vi "陀螺仪.vi"() -> ()   [LabVIEW 2017]
uses:
  <vilib>/myRIO/Instrument Drivers/Onboard IO/I2C/typedefs/I2C User Configuration.ctl
  <vilib>/myRIO/Instrument Drivers/Onboard IO/I2C/typedefs/I2C Transfer Rate.ctl
  <vilib>/Platform/TimedLoop/XDataNode/timing_clust.ctl
  <vilib>/Platform/TimedLoop/XDataNode/nitl_modes.ctl
  <vilib>/Platform/TimedLoop/XDataNode/wakeup.ctl
  <vilib>/myRIO/Instrument Drivers/Onboard IO/I2C/typedefs/I2C Reference.ctl
  <vilib>/myRIO/Common/Instrument Driver Framework/Utilities/typedefs/myRIO Generic Hardware Reference.ctl
  <vilib>/myRIO/Common/Instrument Driver Framework/Utilities/typedefs/Hardware Version Enum.ctl
  <vilib>/myRIO/Common/Instrument Driver Framework/Utilities/typedefs/myRIO v1.0 Reference.ctl
  <vilib>/myRIO/Common/Instrument Driver Framework/Utilities/typedefs/Generic FPGA Reference.ctl
  <vilib>/myRIO/Common/Instrument Driver Framework/myRIO v1.0/I2C/typedefs/I2C Channels Enum.ctl
  <vilib>/myRIO/Instrument Drivers/Onboard IO/I2C/typedefs/I2C Configuration.ctl
  <vilib>/userdefined/High Color/nirio_resource_hc.ctl
  <vilib>/myRIO/Common/Instrument Driver Framework/myRIO v1.0/I2C/vis/myRIO v1.1 Open I2C.vi
  <vilib>/myRIO/Common/Instrument Driver Framework/Utilities/vis/Validate Channels.vi
  <vilib>/myRIO/Common/Instrument Driver Framework/myRIO v1.0/I2C/vis/myRIO v1.0 Reserve I2C.vi
  <vilib>/myRIO/Common/Instrument Driver Framework/myRIO v1.0/UART/vis/myRIO v1.0 Close UART.vi
  <vilib>/myRIO/Common/Instrument Driver Framework/myRIO v1.0/I2C/vis/myRIO v1.0 Build MUX Configuration I2C.vi
  <vilib>/myRIO/Common/Instrument Driver Framework/myRIO v1.0/Resource Manager/vis/myRIO v1.0 Reserve Channel List.vi
  <vilib>/myRIO/Common/Instrument Driver Framework/myRIO v1.0/Resource Manager/vis/myRIO v1.0 Create Configuration List.vi
  <vilib>/myRIO/Common/Instrument Driver Framework/myRIO v1.0/Resource Manager/vis/myRIO v1.0 Reserve Channel.vi
  <vilib>/myRIO/Common/Instrument Driver Framework/myRIO v1.0/Resource Manager/vis/myRIO v1.0 Unreserve Channel.vi
  <vilib>/myRIO/Common/Instrument Driver Framework/myRIO v1.0/Resource Manager/vis/myRIO v1.0 Build Mutex Name.vi
  <vilib>/Utility/VariantDataType/GetNumericInfo.vi
  <vilib>/Utility/error.llb/Error Cluster From Error Code.vi
  <vilib>/myRIO/Common/Instrument Driver Framework/myRIO v1.0/myRIO v1.1 Open.vi
  <vilib>/myRIO/Common/Instrument Driver Framework/Utilities/vis/IO Manager.vi
  <vilib>/myRIO/Common/Instrument Driver Framework/Utilities/vis/Configuration Manager.vi
  <vilib>/myRIO/Common/Instrument Driver Framework/myRIO v1.0/Resource Manager/vis/myRIO v1.0 Configure IO.vi
  <vilib>/myRIO/Common/Instrument Driver Framework/myRIO v1.0/myRIO v1.0 Close.vi
  <vilib>/myRIO/Common/Instrument Driver Framework/myRIO v1.0/I2C/vis/myRIO v1.0 Configure I2C.vi
  <vilib>/myRIO/Common/Instrument Driver Framework/myRIO v1.0/I2C/vis/myRIO v1.0 Write I2C.vi
  <vilib>/myRIO/Common/Instrument Driver Framework/myRIO v1.0/I2C/vis/myRIO v1.0 Read I2C.vi
  <vilib>/myRIO/Common/Instrument Driver Framework/Utilities/vis/FPGA Ref Manager.vi
  <vilib>/myRIO/Common/Instrument Driver Framework/myRIO v1.0/myRIO v1.0 Reset FPGA.vi
  <vilib>/myRIO/Common/Instrument Driver Framework/myRIO v1.0/IRQ/vis/myRIO v1.0 IRQ Info FGV.vi
  <vilib>/myRIO/Common/Instrument Driver Framework/myRIO v1.0/IRQ/vis/myRIO v1.0 Timer IRQ Info FGV.vi
  <vilib>/myRIO/Common/Instrument Driver Framework/myRIO v1.0/IRQ/vis/myRIO v1.0 ISR Agent.vi
  <vilib>/myRIO/Instrument Drivers/Onboard IO/I2C/vis/myRIO I2C Open.xnode
  <vilib>/Platform/TimedLoop/XDataNode/XDataNode.xnode
  <vilib>/myRIO/Instrument Drivers/Onboard IO/I2C/I2C.lvlib
  <vilib>/ptbypt/NI_PtbyPt.lvlib
  <vilib>/Platform/TimedLoop/XDataNode/XDNodeRunTimeDep.lvlib
  <vilib>/myRIO/Instrument Drivers/Utilities/Utilities.lvlib
panel:
  in  "y":dbl=26.5
  in  "x":dbl=-16.0
  in  "initialize":bool caption="初始化"
  in  "停止":bool
  out "加速度":cluster{i16, i16, i16}(graph)
  out "角度":T1(graph)
  out "角速度":cluster{"x":dbl, dbl, dbl}(graph)
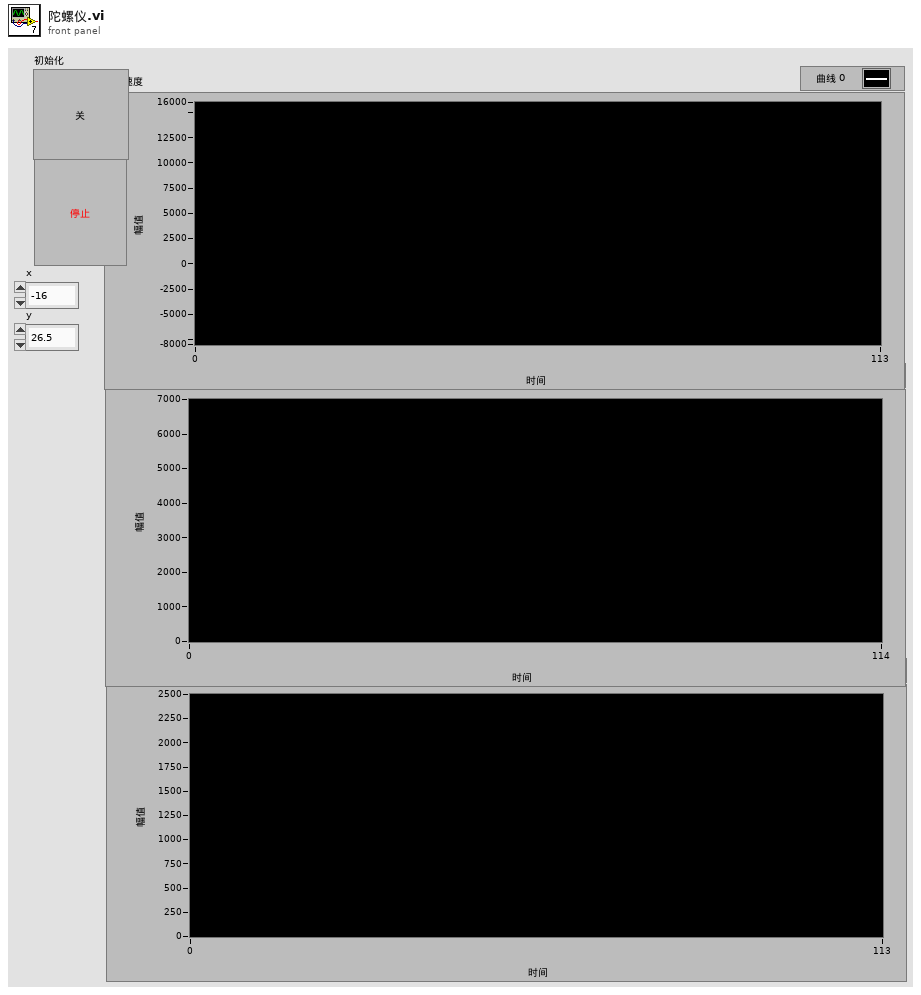
[diagram p1: front panel]
types:
  T1 = cluster{"integral x(t)":dbl, "integral x(t)":dbl, "integral x(t)":dbl}
  T2 = typedef "I2C.lvlib/I2C User Configuration.ctl" = cluster{"I2C Transfer Rate":T3}
  T3 = typedef "I2C.lvlib/I2C Transfer Rate.ctl" = enum16{"Standard mode (100 kbps)", "Fast mode (400 kbps)"}
  T4 = typedef "I2C.lvlib/I2C Reference.ctl" = cluster{"myRIO Reference":T5, "I2C Channels Enum":T9, "I2C Configuration":T10}
  T5 = typedef "myRIO Generic Hardware Reference.ctl" = cluster{"myRIO Model":T6, "myRIO Hardware Reference":T7}
  T6 = typedef "Hardware Version Enum.ctl" = enum16{"Unknown", "myRIO-1900", "myRIO-1950", "roboRIO", "NI ELVIS RIO CM"}
  T7 = typedef "myRIO v1.0 Reference.ctl" = cluster{"Generic FPGA Reference":T8, "Allow multiple opens":bool}
  T8 = typedef "Generic FPGA Reference.ctl" = refnum<k20>
  T9 = typedef "I2C Channels Enum.ctl" = enum16{"Not Connected", "A/I2C", "B/I2C", "I2C/I2C"}
  T10 = typedef "I2C.lvlib/I2C Configuration.ctl" = cluster{"I2C Transfer Rate":T3}
  T11 = typedef "XDNodeRunTimeDep.lvlib/timing_clust.ctl" = cluster{"Expected End [f-1]":u64, "Actual End [f-1]":u64, "Finished Late? [f-1]":bool, "Expected End [i-1]":u64, "Actual End [i-1]":u64, "Finished Late? [i-1]":bool, "Expected Start [i]":u64, "Actual Start [i]":u64, "Expected Start [f]":u64, "Actual Start [f]":u64, "Source Name":string, "Structure Name":string, "Period":i64, "Deadline":i64, "Offset":i64, "Start":i64, "Priority":i32, "Timeout":i32, "Mode":T12, "Wakeup Reason":T13, "Error":errorcluster, "Source Type":string, "Secondary Source Type":string, "Global End Time":u64, "Global Start Time":u64, "Frame Duration":u64, "Iteration Duration":u64, "Assigned CPU":i32, "I/O Scan Engine Mode":u32}
  T12 = typedef "XDNodeRunTimeDep.lvlib/nitl_modes.ctl" = enum32{"No Change", "Process missed periods, maintain original phase", "Discard missed periods, maintain original phase", "Process missed periods, ignore original phase", "Discard missed periods, ignore original phase"}
  T13 = typedef "XDNodeRunTimeDep.lvlib/wakeup.ctl" = enum32{"Normal", "Aborted", "Asynchronous wakeup", "Timing source error", "Timed loop error", "Timeout"}
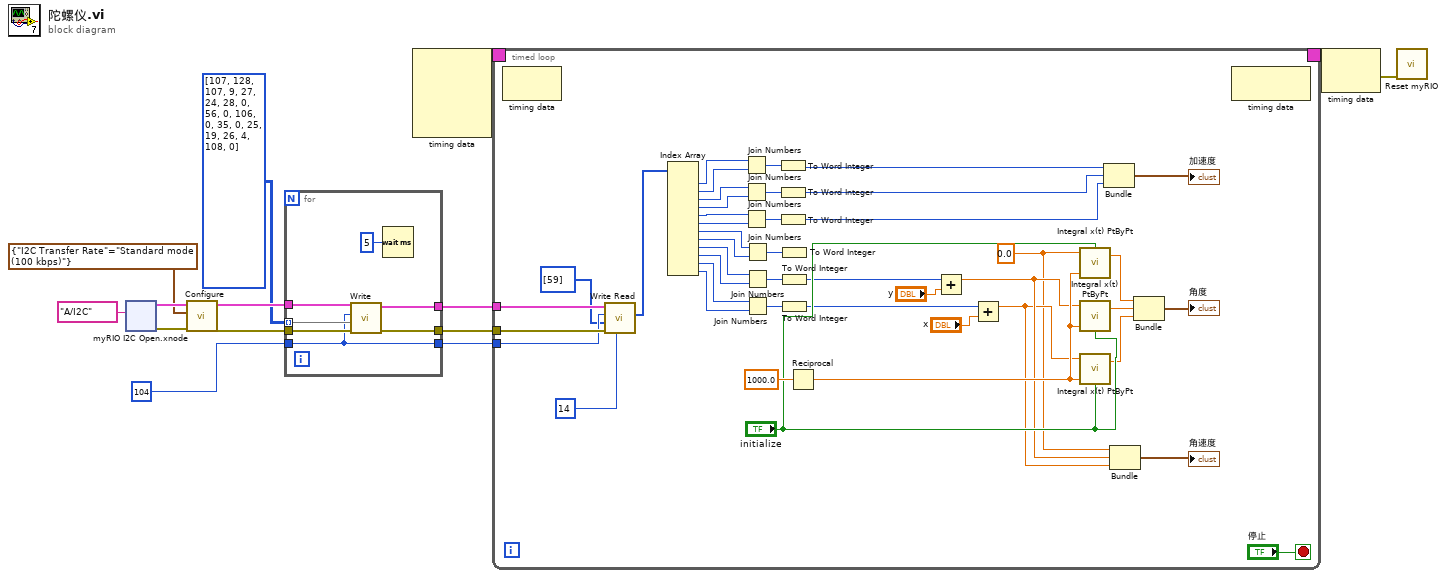
[diagram p0: block diagram]
diagram:
  n1 = xnode "myRIO I2C Open.xnode"("Channel Name"=tag "A/I2C") -> ("error out"=w14:errorcluster, "I2C Ref Out"=w13:T4)  [unwired: 2 in]
  n2 = call <vilib>:"Configure.vi"("error in (no error)"=w14, "I2C User Configuration"=T2 {"I2C Transfer Rate"=enum."Standard mode (100 kbps)"}, "I2C Ref In"=w13) -> ("error out"=w9:errorcluster, "I2C Ref Out"=w10:T4)  [unwired: 7 in]
  n3 = for {
    tunnel: w10 -> [w21]
    tunnel: w9 -> [w20]
    tunnel: [w19] -> w8
    tunnel: [w18] -> w7
    tunnel: u8 104 ("Slave Address (7-bit)") -> [w15]
    tunnel: u8[][] [[107, 128], [107, 9], [27, 24], [28, 0], [56, 0], [106, 0], [35, 0], [25, 19], [26, 4], [108, 0]] ("Bytes to Write") -> [w16] mode=indexing
    tunnel: [w15] -> w4
    n4 = call <vilib>:"Write.vi"("error in (no error)"=w20, "Bytes to Write"=w16, "Slave Address (7-bit)"=w15, "I2C Ref In"=w21) -> ("error out"=w18:errorcluster, "I2C Ref Out"=w19:T4)  [unwired: 6 in]
    n5 = Wait (ms)(milliseconds to wait=u32 5 ("等待时间（毫秒）")) -> ()  [unwired: 1 out]
  }
  n6 = node-c288() -> (w3:T11)  [unwired: 4 in]
  n7 = timed-loop {
    timing: w3 -> [_]
    timing-out: [_] -> w2
    tunnel: w8 -> [w65]
    tunnel: w7 -> [w64]
    tunnel: w4 -> [w63]
    stop <- "停止" stop-if-true
    w22 = 0.0 ("x")
    n8 = node-c288() -> ()  [unwired: 1 in, 1 out]
    n9 = call <vilib>:"Write Read.vi"("Byte Count"=u32 14, "error in (no error)"=w64, "Bytes to Write"=u8[] [59], "Slave Address (7-bit)"=w63, "I2C Ref In"=w65) -> ("Bytes Read"=w61:u8[])  [unwired: 3 in, 2 out]
    n10 = Index Array(array=w61) -> (element #1=w60:u8, element #2=w59:u8, element #3=w58:u8, element #4=w57:u8, element #5=w56:u8, element #6=w55:u8, element #7=w54:u8, element #8=w53:u8, element #9=w52:u8, element #10=w51:u8, element #11=w50:u8, element #12=w49:u8)  [unwired: 12 in]
    n11 = Join Numbers(hi=w60, lo=w59) -> ((hi.lo)=w47:u16)
    n12 = Join Numbers(hi=w58, lo=w57) -> ((hi.lo)=w46:u16)
    n13 = Join Numbers(hi=w56, lo=w55) -> ((hi.lo)=w45:u16)
    n14 = Join Numbers(hi=w54, lo=w53) -> ((hi.lo)=w44:u16)
    n15 = Join Numbers(hi=w52, lo=w51) -> ((hi.lo)=w43:u16)
    n16 = Join Numbers(hi=w50, lo=w49) -> ((hi.lo)=w42:u16)
    n17 = To Word Integer(number=w47) -> (16bit integer=w41:i16)
    n18 = To Word Integer(number=w46) -> (16bit integer=w40:i16)
    n19 = To Word Integer(number=w45) -> (16bit integer=w39:i16)
    n20 = To Word Integer(number=w44) -> ()  [unwired: 1 out]
    n21 = To Word Integer(number=w43) -> (16bit integer=w28:i16)
    n22 = To Word Integer(number=w42) -> (16bit integer=w27:i16)
    n23 = Reciprocal(x=1000.0) -> (1/x=w37:dbl)
    n24 = Add(x=w28, y="y") -> (x+y=w26:dbl)
    n25 = Add(x=w27, y="x") -> (x+y=w24:dbl)
    n26 = call <vilib>:"Integral x(t) PtByPt.vi"("initialize"="initialize", "dt"=w37, "x"=w22) -> ("integral x(t)"=w35:dbl)  [unwired: 1 in, 1 out]
    n27 = call <vilib>:"Integral x(t) PtByPt.vi"("initialize"="initialize", "dt"=w37, "x"=w26) -> ("integral x(t)"=w34:dbl)  [unwired: 1 in, 1 out]
    n28 = call <vilib>:"Integral x(t) PtByPt.vi"("initialize"="initialize", "dt"=w37, "x"=w24) -> ("integral x(t)"=w29:dbl)  [unwired: 1 in, 1 out]
    n29 = Bundle(w41, w40, w39) -> (→"加速度":cluster{i16, i16, i16})  [unwired: 1 in]
    n30 = Bundle("x"=w22, w26, w24) -> (→"角速度":cluster{"x":dbl, dbl, dbl})  [unwired: 1 in]
    n31 = Bundle("integral x(t)"=w35, "integral x(t)"=w34, "integral x(t)"=w29) -> (→"角度":T1)  [unwired: 1 in]
    n32 = node-c288() -> ()  [unwired: 1 in, 1 out]
  }
  n33 = node-c288(w2) -> (w1:errorcluster)
  n34 = call <vilib>:"Reset myRIO.vi"("error in (no error)"=w1) -> ()  [unwired: 10 in, 1 out]
